vi "GenAxis.vi"(4 "Points2":i32=10, 5 "Plane":u16(ring)=2 items=["X-Y", "Y-Z", "Z-X"], 6 "Plane dimensions (cm)":cluster{"x":dbl, "y":dbl, "z":dbl}={"x"=4.0, "y"=4.0, "z"=4.0} {"x" format="%.2f"; "z" format="%.2f"; "y" format="%.2f"}, 7 "Points1":i32=10) -> (0 "outer index":dbl[](array[numeric]) format="%.2f", 1 "inner index":dbl[](array[numeric]) format="%.2f", 2 "fixed plane":dbl format="%.2f")   [LabVIEW 2022 SP3]
panel:
  out "Waveform Graph 2":dbl[](graph)
  out "Waveform Graph":dbl[](graph)
  # "y\ny\nz"
  # "x\nz\nx"
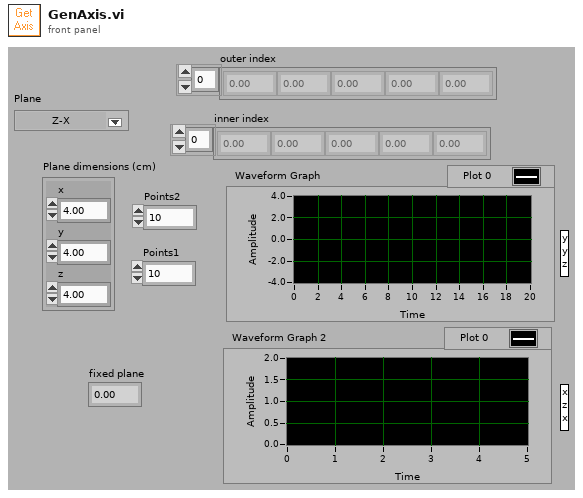
[diagram p1: front panel]
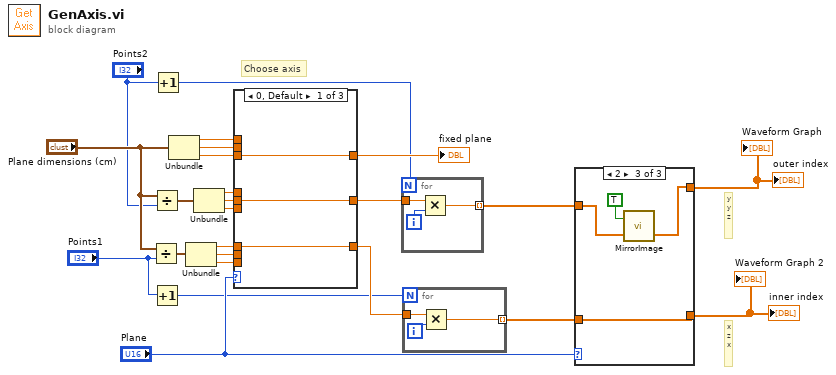
[diagram p0: block diagram]
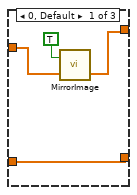
[diagram p2: hidden frame]
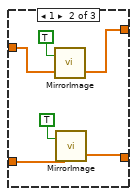
[diagram p3: hidden frame]
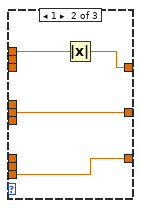
[diagram p4: hidden frame]
diagram:
  # "x\nz\nx"
  # "y\ny\nz"
  # "Choose axis"
  n1 = Divide(x="Plane dimensions (cm)", y="Points1") -> (x/y=w9:cluster{"x":dbl, "y":dbl, "z":dbl})
  n2 = Divide(x="Plane dimensions (cm)", y="Points2") -> (x/y=w22:cluster{"x":dbl, "y":dbl, "z":dbl})
  n3 = Increment(x="Points1") -> (x+1=w2:i32)
  n4 = Increment(x="Points2") -> (x+1=w1:i32)
  n5 = Unbundle("Plane dimensions (cm)") -> ("x"=w24:dbl, "y"=w13:dbl, "z"=w23:dbl)
  n6 = Unbundle(w9) -> ("x"=w5:dbl, "y"=w3:dbl, "z"=w4:dbl)
  n7 = Unbundle(w22) -> ("x"=w21:dbl, "y"=w20:dbl, "z"=w19:dbl)
  n8 = case shown="0, Default" "Plane" {
    tunnel: w24 -> [_ w31 _]
    tunnel: w13 -> [_ _ w34]
    tunnel: w23 -> [w26 _ _]
    tunnel: [w25 w28 w32] -> w17
    tunnel: w21 -> [_ _ _]
    tunnel: [w27 w30 w33] -> w18
    tunnel: w20 -> [w27 w30 _]
    tunnel: [w26 w29 w34] -> w16
    tunnel: w19 -> [_ _ w33]
    tunnel: w5 -> [w25 _ w32]
    tunnel: w4 -> [_ w28 _]
    tunnel: w3 -> [_ _ _]
    frame 0, Default {
    }
    frame 1 {
      n9 = Absolute Value(x=w31) -> (abs(x)=w29:dbl)
    }
    frame 2 {
    }
  }
  "fixed plane" <- w16
  n10 = for {
    N: w1 -> [_]
    tunnel: w18 -> [w36]
    tunnel: [w35] -> w11 mode=indexing
    i -> [w37]
    n11 = Multiply(x=w36, y=w37) -> (x*y=w35:dbl)
  }
  n12 = for {
    N: w2 -> [_]
    tunnel: w17 -> [w39]
    tunnel: [w38] -> w14 mode=indexing
    i -> [w40]
    n13 = Multiply(x=w39, y=w40) -> (x*y=w38:dbl)
  }
  n14 = case shown="2" "Plane" {
    tunnel: w14 -> [w41 w50 w53]
    tunnel: [w41 w48 w53] -> w12
    tunnel: w11 -> [w43 w46 w52]
    tunnel: [w42 w45 w51] -> w10
    frame 0, Default {
      n15 = call "MirrorImage.vi"("input"=w43, "neg?"=TRUE) -> ("output"=w42:dbl[])  [unwired: 1 out]
    }
    frame 1 {
      n16 = call "MirrorImage.vi"("input"=w46, "neg?"=TRUE) -> ("output"=w45:dbl[])  [unwired: 1 out]
      n17 = call "MirrorImage.vi"("input"=w50, "neg?"=TRUE) -> ("output"=w48:dbl[])  [unwired: 1 out]
    }
    frame 2 {
      n18 = call "MirrorImage.vi"("input"=w52, "neg?"=TRUE) -> ("output"=w51:dbl[])  [unwired: 1 out]
    }
  }
  "outer index" <- w10
  "Waveform Graph 2" <- w12
  "Waveform Graph" <- w10
  "inner index" <- w12
